vi "GetSet Visa ressource name.vi"(0 "VISA resource name  in":refnum<visa-resource-name>, 7 "Get/Set":enum16{"Get", "Set"}(ring)=enum."Set", 11 "error in (no error)":errorcluster) -> (4 "VISA resource name out":refnum<visa-resource-name>, 15 "error out":errorcluster)   [LabVIEW 2024, in "GRBL 1.1.lvlib"]
doc: "Set serial port name to the selected controller"
uses:
  GRBL 1.1.lvlib
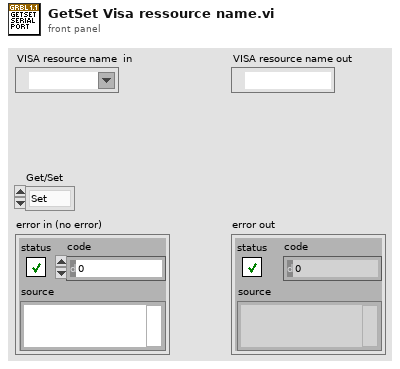
[diagram p1: front panel]
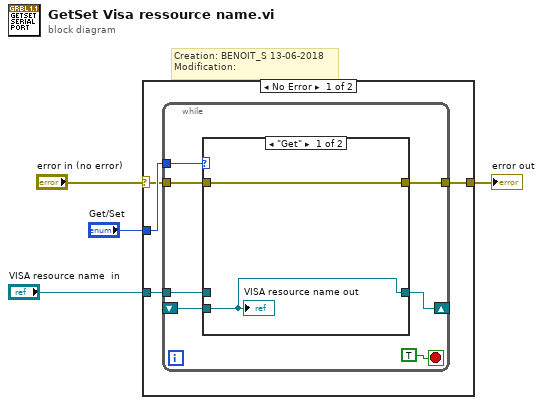
[diagram p0: block diagram]
diagram:
  # "Creation: BENOIT_S 13-06-2018\nModification:"
  n1 = case shown="No Error" "error in (no error)" {
    selector: "error in (no error)" -> [w6 w20]
    tunnel: [w5 w20] -> w3
    tunnel: "Get/Set" -> [w8 _]
    tunnel: "VISA resource name  in" -> [w7 _]
    frame No Error {
      n2 = while {
        tunnel: w8 -> [w14]
        shift-right: [w13] -> _
        shift-left: _ -> [w12]
        tunnel: w7 -> [w11]
        tunnel: w6 -> [w10]
        tunnel: [w9] -> w5
        stop <- TRUE stop-if-true
        n3 = case shown="\"Get\"" w14 {
          tunnel: [w16 w18] -> w13
          tunnel: w12 -> [w16 _]
          tunnel: w11 -> [_ w18]
          tunnel: w10 -> [w17 w19]
          tunnel: [w17 w19] -> w9
          frame "Get" {
            "VISA resource name out" <- w16
          }
          frame "Set" {
          }
        }
      }
    }
    frame Error {
    }
  }
  "error out" <- w3
